vi "svfa_Next Good FFT Size.vi"(1 "FFT Size":i32) -> (0 "least bigger good size":i32)   [LabVIEW 2017]
panel:
  # "This VI returns the least bigger number contains prime factors all less than 13"
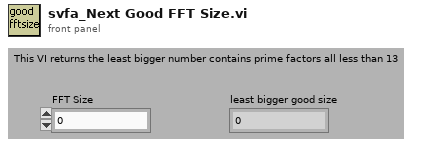
[diagram p1: front panel]
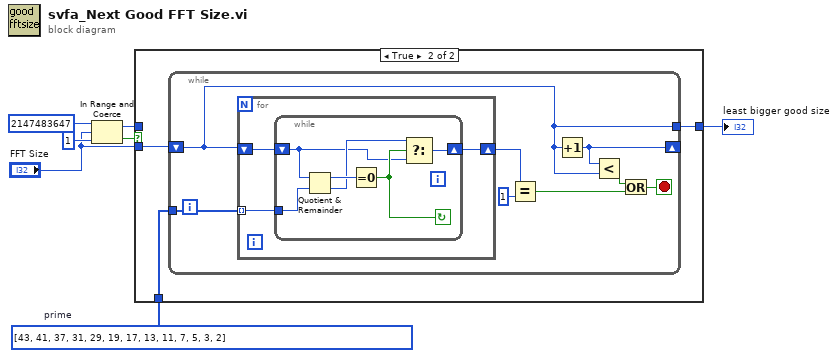
[diagram p0: block diagram]
diagram:
  w6 = i32[] [43, 41, 37, 31, 29, 19, 17, 13, 11, 7, 5, 3, 2]  # prime
  n1 = In Range and Coerce(upper limit=2147483647, x="FFT Size", lower limit=1) -> (coerced(x)=w1:i32, In Range?=w2:bool)
  n2 = case shown="True" w2 {
    tunnel: "FFT Size" -> [_ w11]
    tunnel: [w8 w10] -> w7
    tunnel: w6 -> [_ w9]
    tunnel: w1 -> [w8 _]
    frame False {
    }
    frame True {
      n3 = while {
        tunnel: [w15] -> w10
        tunnel: w9 -> [w19]
        shift-left: w11 -> [w15]
        shift-right: [w16] -> _
        stop <- w12 stop-if-true
        n4 = for {
          tunnel: w19 -> [w22] mode=indexing
          shift-right: [w20] -> w17
          shift-left: w15 -> [w21]
          n5 = while {
            shift-left: w21 -> [w24]
            shift-right: [w27] -> w20
            tunnel: w22 -> [w23]
            stop <- w26 continue-if-true
            n6 = Quotient & Remainder(x=w24, y=w23) -> (x-y*floor(x/y)=w28:i32, floor(x/y)=w25:i32)
            n7 = Equal To 0?(x=w28) -> (x = 0?=w26:bool)
            n8 = Select(t=w25, s=w26, f=w24) -> (s? t:f=w27:i32)
          }
        }
        n9 = Equal?(x=w17, y=1) -> (x = y?=w13:bool)
        n10 = Increment(x=w15) -> (x+1=w16:i32)
        n11 = Less?(x=w16, y=w15) -> (x < y?=w14:bool)
        n12 = Or(x=w14, y=w13) -> (x .or. y?=w12:bool)
      }
    }
  }
  "least bigger good size" <- w7
